vi "Pick_Vitreous.vi"() -> ()   [LabVIEW 2022 SP3]
uses:
  ViewData/-ReadEye/Header.ctl
  ViewData/-ReadEye/TypeDefs/TypeofMean.ctl
  <vilib>/Utility/file.llb/Write Delimited Spreadsheet (string).vi
  <vilib>/Utility/file.llb/Write Delimited Spreadsheet (I64).vi
  <vilib>/Analysis/NI_AALPro.lvlib
panel:
  out "RF":dbl[](graph)
  out "x/y":dbl
  in  "dB":dbl(slide)=-50.20408163265306 scale=0.0..255.0
  out "Waveform Graph":dbl[](graph)
  out "Transducer":u16(ring)=1500 items=["Aviso B10/B15"=1024, "B15 Orbit/Long Vitreous (60 mm)"=1500, "B15 Eye/Vitreous (40 mm)"=2133, "Annular Array"=3282, "Annular Array"=3362, "Lin50"=1000]
  in  "File Params?":bool=TRUE
  out "inc x (mm)":dbl format="%.3f"
  out "inc y (mm)":dbl format="%.3f"
  out "Sector view":dbl[][](graph)
  in  "Pixels in x":i16=256
  in  "Pixels in y":i16=489
  in  "Create EYE batch":bool
  in  "Save Comment ?":bool
  in  "Comment Field (Optional)":string
  in  "Good Case":bool
  in  "Current Image #":i32(slide) min=0 max=134 step=1 scale=0.0..7.0
  in  "stop":bool
  in  "File to Process":path=path "Select a file."
  out "Raw Image File":dbl[][](graph)
  in  "RF lines":i32=170
  in  "RF pts":i32=1024
  out "Total Raw File Size":i32
  out "# Images":dbl
  # "For screening *.raw and *.rf  stacks from Quantel Machines. Attempts to extract info from file name but may need to modify parameters"
  # "Image Parameters"
  # "These remain static!!!"
  # "Push folder symbol (above) to select raw data file to process\nPress \"Page Up\" on keybard to increment up one image\nPress \"Page Down\" on keyboard to decrement down one image\nPress \"ESC\" on keyboard to log number of good image\nSelect \"Save Comment\" to save any text that is entered into \"Comment Field\"\nExit program by pressing \"Stop\""
  # "-\tFor 20MHz, the sampling rate is 60MHz,\n-\tFor 15MHz, depending of the mode:\no\tFor Orbit and Long Vitreous (image displayed with 60mm), the sampling frequency is 20MHz,\no\tFor Eye and Vitreous, (image displayed with 40mm), the sampling frequency is 40MHz\n-\tFor 50MHz, the sampling rate is 80MHz,"
  # "Select  \"Show Context Help\" under \"Help\" menu and scroll over control to see a brief description in pop-up window."
  # "© 2022 Weill Cornell Medicine"
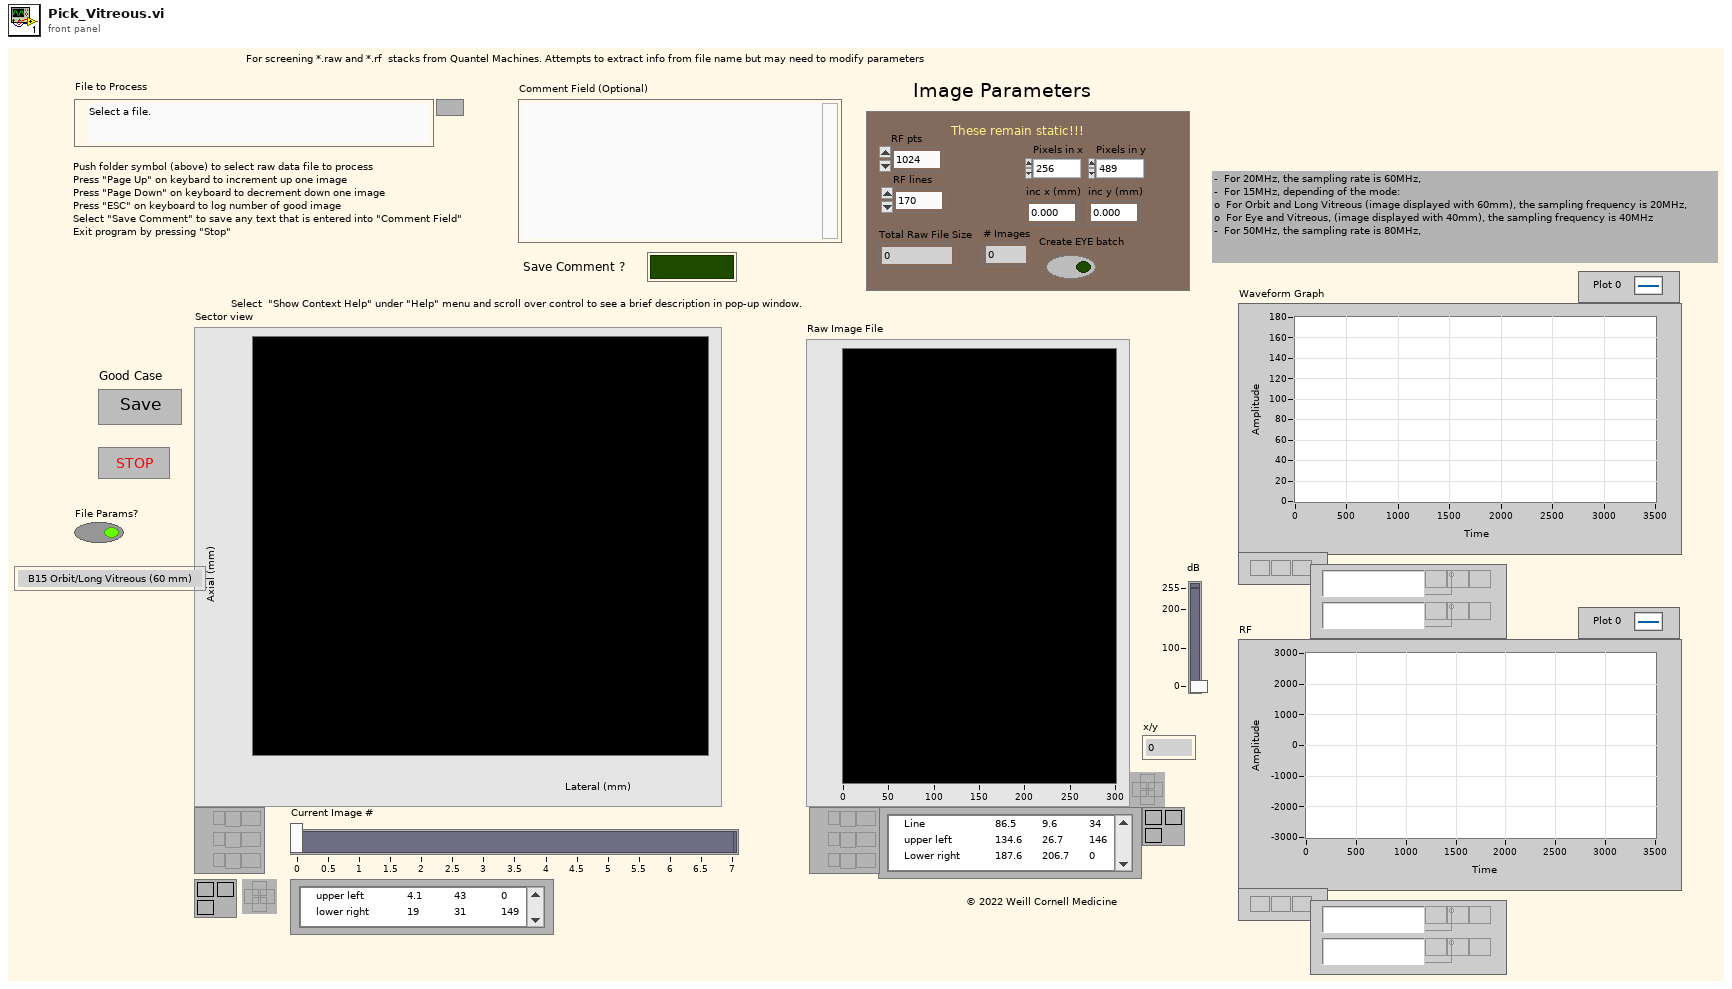
[diagram p1: front panel]
types:
  T1 = typedef "Header.ctl" = cluster{"header info":cluster{"Header":string, "Head length":i16}, "A/D info":cluster{"# rf points per line":u16, "# lines per scan":u16, "sample rate MHz":u16, "# A/D bits":i16, "# bytes per A/D":u16, "TGC Flag":u16, "A/D Type":string}, "Tranducer Info":cluster{"bandwidth":sgl, "center freq":sgl, "start freq":sgl, "ID":i32}, "Scan Info":cluster{"delay":sgl, "pivot distance":sgl, "sector scan angle":sgl, "operator":string, "Scan Mode":string, "location":string}, "Time/Date Info":cluster{"date":string, "time":string}, "RF Info":cluster{"RF file name":string, "RF file att":string, "RF cal file name":string, "RF cal file att":string}, "Patient Info":cluster{"ID":string, "extended ID":string, "age":u16, "sex":string, "previously\nscanned":string, "PSA":sgl, "LOS":u8, "Ethnicty 2":u8, "Race":u8}, "Tissue Type":cluster{"organ":i16, "disease type":i16, "disease location":i16, "IQ_pts":u16, "RcvBuffer":u8, "RcvFrame":u16, "IQBuff":u8, "IQFrame":u16, "IQPage":u8}, "Votage scaling":cluster{"Digitizer (dB)":sgl, "Gain (dB)":sgl, "Atten (dB)":sgl}, "Comment":string, "Misc Info":cluster{"avg num":u16, "c speed":i16, "Div By or SF zones":i16, "XMIT CHS":u8, "RCV CHS":u8, "Xmit angle":sgl}, "Therapy Parameters":cluster{"Theraputic Freq (MHz)":sgl, "Time on (s)":sgl, "Therapy amplitude (mV)":sgl, "Lines Before":u16, "Lines After":u16}, "Scan Settings":cluster{"Energy (uJ or V)":u8, "Damp (Ohm) or Fc":u8, "HP Filt (KHz)":u8, "LP Filt (MHz)":u8, "Gain (db)":u8, "prf (kHz)":sgl, "Distance between\nscan lines (um)":u16, "Distance between\nscan planes (um)":u16, "Scan line gap (um)":sgl, "Scan plane gap (um)":sgl}, "Compression Parameters":cluster{"F1 (MHz)":sgl, "F2 (MHz)":sgl, "% taper":sgl, "duration":sgl}, "Patient Info Xtra":cluster{"First Name":string, "Last Name":string, "Notes":string}, "ROI Box":u16[]}
  T2 = cluster{"low cutoff":i32, "order":i32, "high cutoff":i32}
  T3 = typedef "TypeofMean.ctl" = enum16{"Mean from lines", "Mean just lines", "Poly Mean", "No mean", "Filter"}
  T4 = enum16{"open", "replace", "create", "open or create", "replace or create", "replace or create with confirmation"}
  T5 = cluster{"Frames":i32, "RF Points":i32, "RF lines":i32, "Month":string, "Day":i32, "Year":i32, "Case":string, "data format":string}
  T6 = cluster{"delay":sgl, "pivot distance":sgl, "sector scan angle":sgl, "operator":string, "Scan Mode":string, "location":string}
  T7 = cluster{"X right":dbl, "X left":dbl, "Y low":dbl, "Y high":dbl}
  T8 = typedef "LVPointDoubleTypeDef.ctl" = cluster{"Cursor X":dbl, "Cursor Y":dbl}
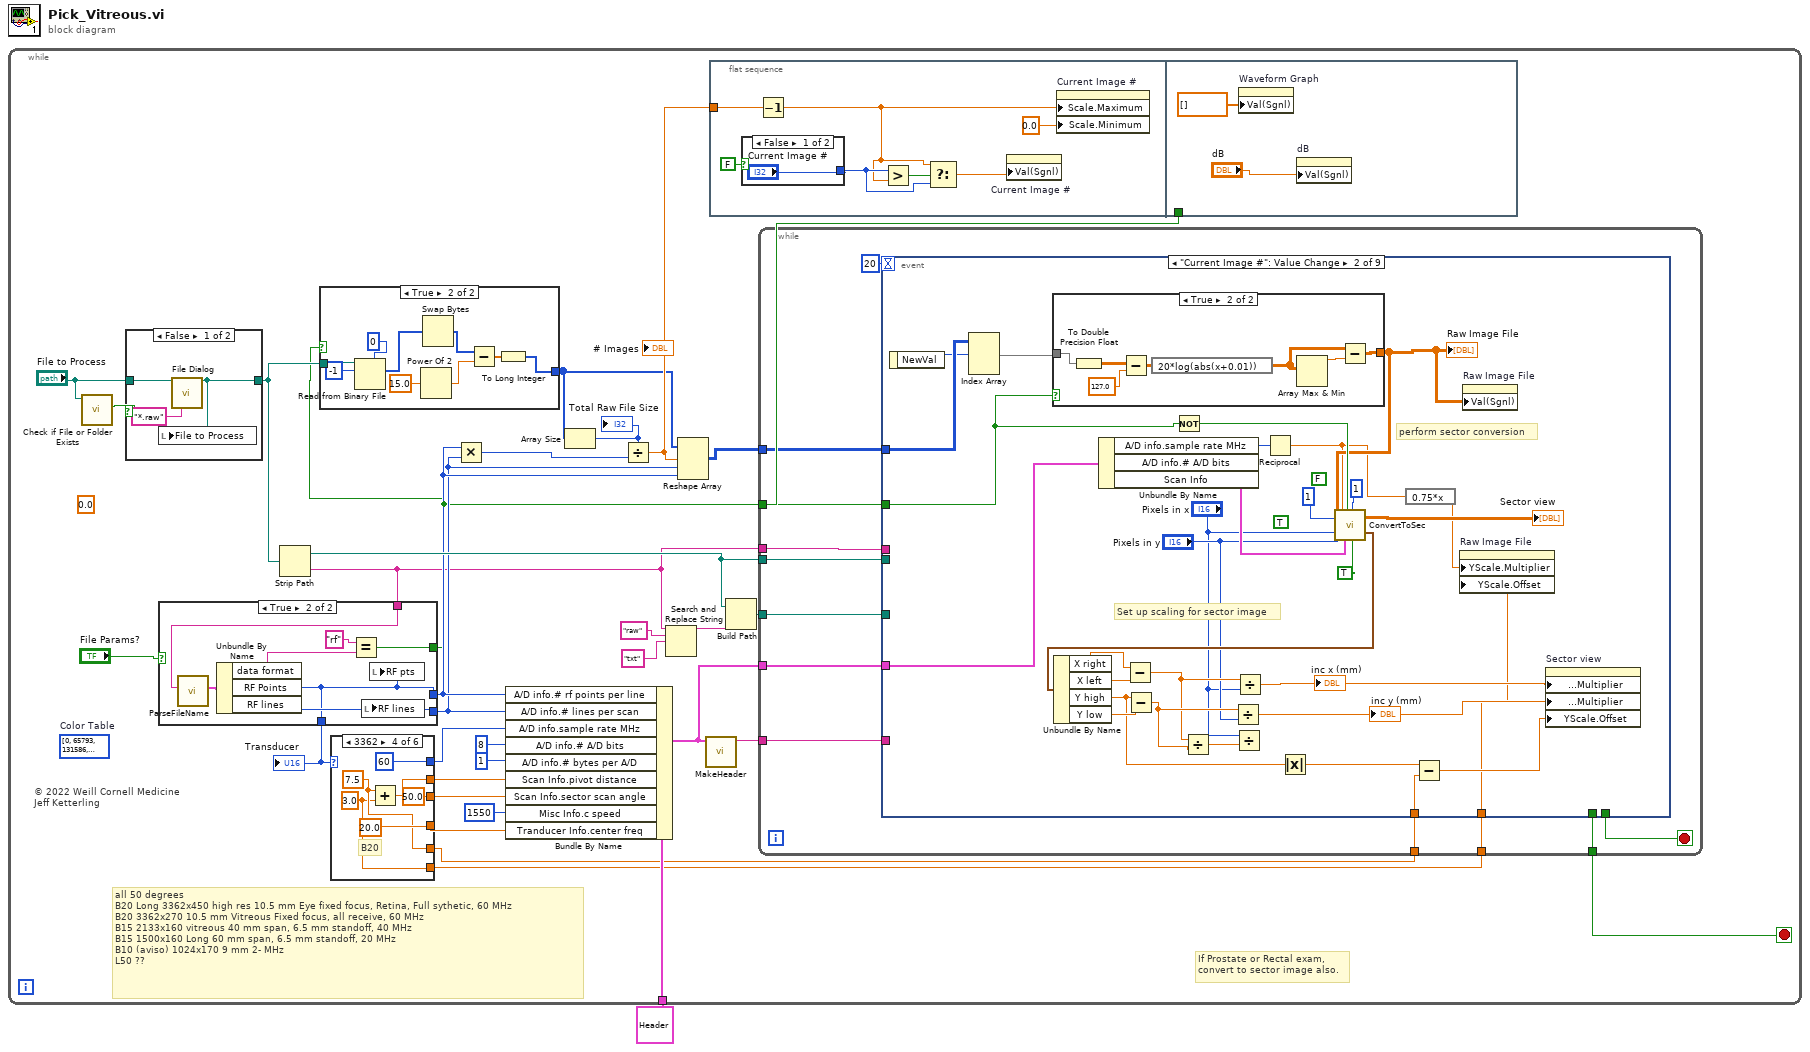
[diagram p0: block diagram]
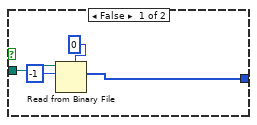
[diagram p2: hidden frame]
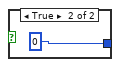
[diagram p3: hidden frame]
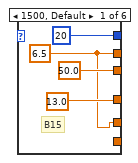
[diagram p4: hidden frame]
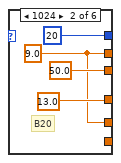
[diagram p5: hidden frame]
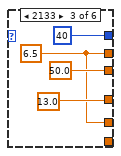
[diagram p6: hidden frame]
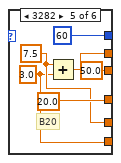
[diagram p7: hidden frame]
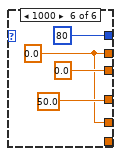
[diagram p8: hidden frame]
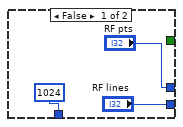
[diagram p9: hidden frame]
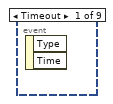
[diagram p11: hidden frame]
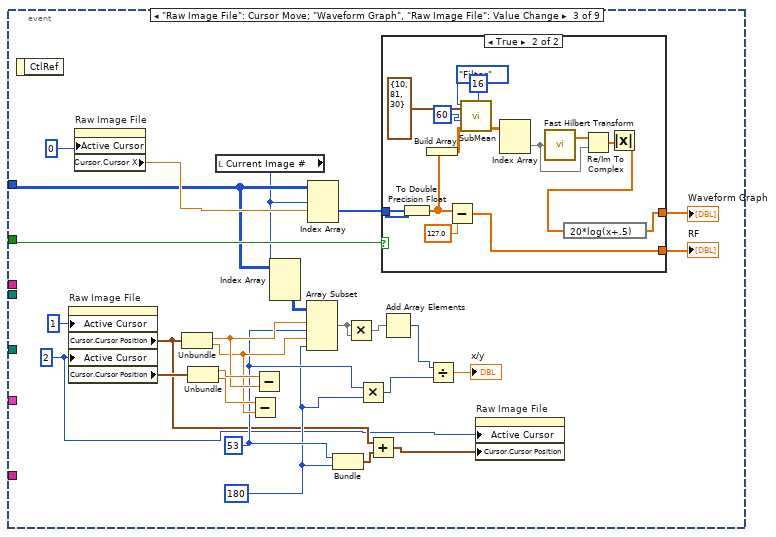
[diagram p13: hidden frame]
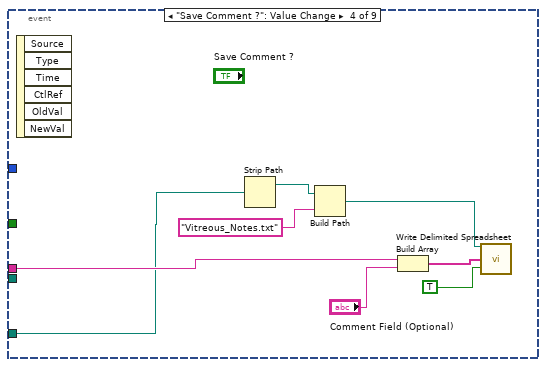
[diagram p15: hidden frame]
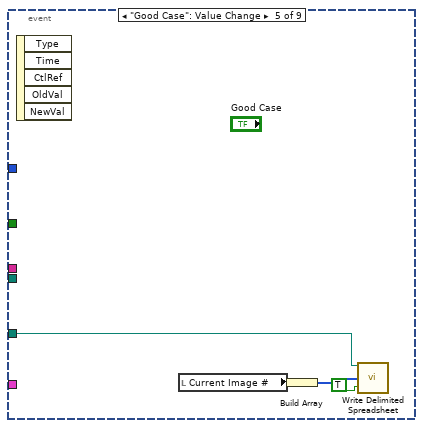
[diagram p16: hidden frame]
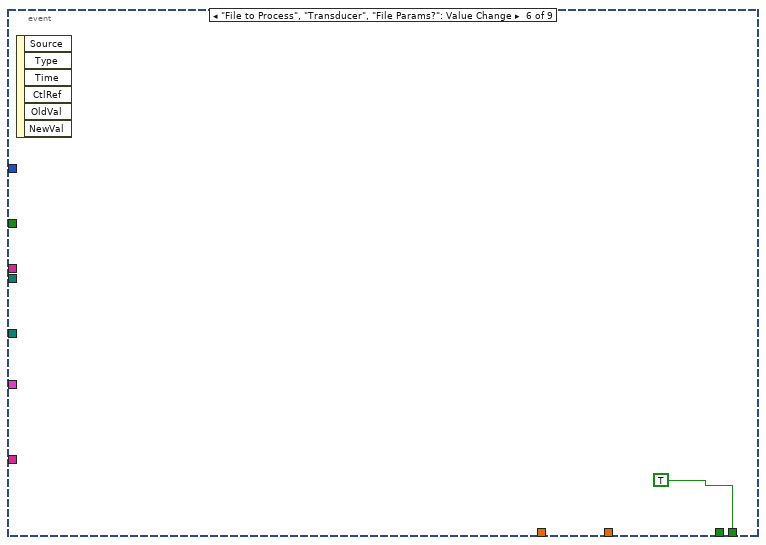
[diagram p17: hidden frame]
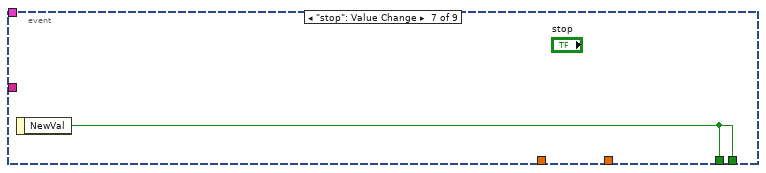
[diagram p18: hidden frame]
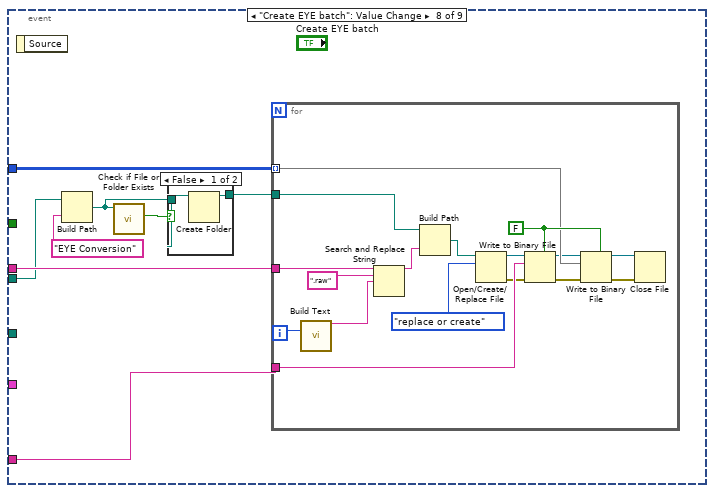
[diagram p19: hidden frame]
diagram:
  n1 = while {
    tunnel: T1 {"header info"={"Header"="", "Head length"=1024}, "A/D info"={"# rf points per line"=0, "# lines per scan"=0, "sample rate MHz"=0, "# A/D bits"=0, "# bytes per A/D"=0, "TGC Flag"=0, "A/D Type"=""}, "Tranducer Info"={"bandwidth"=0.0, "center freq"=0.0, "start freq"=0.0, "ID"=0}, "Scan Info"={"delay"=0.0, "pivot distance"=0.0, "sector scan angle"=0.0, "operator"="", "Scan Mode"="", "location"=""}, "Time/Date Info"={"date"="", "time"=""}, "RF Info"={"RF file name"="", "RF file att"="", "RF cal file name"="", "RF cal file att"=""}, "Patient Info"={"ID"="", "extended ID"="", "age"=0, "sex"="", "previously\nscanned"="", "PSA"=0.0, "LOS"=1, "Ethnicty 2"=3, "Race"=3}, "Tissue Type"={"organ"=0, "disease type"=0, "disease location"=0, "IQ_pts"=0, "RcvBuffer"=0, "RcvFrame"=0, "IQBuff"=0, "IQFrame"=0, "IQPage"=0}, "Votage scaling"={"Digitizer (dB)"=0.0, "Gain (dB)"=0.0, "Atten (dB)"=0.0}, "Comment"="", "Misc Info"={"avg num"=0, "c speed"=0, "Div By or SF zones"=0, "XMIT CHS"=0, "RCV CHS"=0, "Xmit angle"=0.0}, "Therapy Parameters"={"Theraputic Freq (MHz)"=0.1, "Time on (s)"=1.0, "Therapy amplitude (mV)"=50.0, "Lines Before"=20, "Lines After"=80}, "Scan Settings"={"Energy (uJ or V)"=0, "Damp (Ohm) or Fc"=0, "HP Filt (KHz)"=0, "LP Filt (MHz)"=0, "Gain (db)"=0, "prf (kHz)"=0.0, "Distance between\nscan lines (um)"=0, "Distance between\nscan planes (um)"=0, "Scan line gap (um)"=0.0, "Scan plane gap (um)"=0.0}, "Compression Parameters"={"F1 (MHz)"=0.0, "F2 (MHz)"=0.0, "% taper"=0.0, "duration"=0.0}, "Patient Info Xtra"={"First Name"="", "Last Name"="", "Notes"=""}, "ROI Box"=[0, 0, 0, 0]} ("Header In") -> [w25]
    stop <- w30 stop-if-true
    (unwired) u32[] [0, 65793, 131586, 197379, 263172, 328965, 394758, 460551, 526344, 592137, 592137, 657930, 723723, 789516, 855309, 921102, 986895, 1052688, 1118481, 1184274, 1250067, 1315860, 1381653, 1447446, 1513239, 1579032, 1644825, 1710618, 1776411, 1842204, 1907997, 1973790, 2039583, 2105376, 2171169, 2236962, 2302755, 2368548, 2434341, 2500134, 2565927, 2631720, 2697513, 2763306, 2829099, 2894892, 2960685, 3026478, 3092271, 3158064, 3223857, 3289650, 3355443, 3421236, 3487029, 3552822, 3618615, 3684408, 3750201, 3815994, 3881787, 3947580, 4013373, 4079166, 4144959, 4210752, 4276545, 4342338, 4408131, 4473924, 4539717, 4605510, 4671303, 4737096, 4802889, 4868682, 4934475, 5000268, 5066061, 5131854, 5197647, 5263440, 5329233, 5395026, 5460819, 5526612, 5592405, 5658198, 5723991, 5789784, 5855577, 5921370, 5987163, 6052956, 6118749, 6184542, 6250335, 6316128, 6381921, 6447714, 6513507, 6579300, 6645093, 6710886, 6776679, 6842472, 6908265, 6974058, 7039851, 7105644, 7171437, 7237230, 7303023, 7368816, 7434609, 7500402, 7566195, 7631988, 7697781, 7763574, 7829367, 7895160, 7960953, 8026746, 8092539, 8158332, 8224125, 8289918, 8355711, 8421504, 8487297, 8553090, 8618883, 8684676, 8750469, 8816262, 8882055, 8947848, 9013641, 9079434, 9145227, 9211020, 9276813, 9342606, 9408399, 9474192, 9539985, 9605778, 9671571, 9737364, 9803157, 9868950, 9934743, 10000536, 10066329, 10132122, 10197915, 10263708, 10329501, 10395294, 10461087, 10526880, 10592673, 10658466, 10724259, 10790052, 10855845, 10921638, 10987431, 11053224, 11119017, 11184810, 11250603, 11316396, 11382189, 11447982, 11513775, 11579568, 11645361, 11711154, 11776947, 11842740, 11908533, 11974326, 12040119, 12105912, 12171705, 12237498, 12303291, 12369084, 12434877, 12500670, 12566463, 12632256, 12698049, 12763842, 12829635, 12895428, 12961221, 13027014, 13092807, 13158600, 13224393, 13290186, 13355979, 13421772, 13487565, 13553358, 13619151, 13684944, 13750737, 13816530, 13882323, 13948116, 14013909, 14079702, 14145495, 14211288, 14277081, 14342874, 14408667, 14474460, 14540253, 14606046, 14671839, 14737632, 14803425, 14869218, 14935011, 15000804, 15066597, 15132390, 15198183, 15263976, 15329769, 15395562, 15461355, 15527148, 15592941, 15658734, 15724527, 15790320, 15856113, 15921906, 15987699, 16053492, 16119285, 16185078, 16250871, 16316664, 16382457, 16448250, 16514043, 16579836, 16645629, 0]  # Color Table
    (unwired) sgl 0.0 ("Scan Info.pivot distance")
    # "If Prostate or Rectal exam,\nconvert to sector image also."
    # "all 50 degrees\nB20 Long 3362x450 high res 10.5 mm Eye fixed focus, Retina, Full sythetic, 60 MHz\nB20 3362x270 10.5 mm Vitreous Fixed focus, all receive, 60 MHz\nB15 2133x160 vitreous 40 mm span, 6.5 mm standoff, 40 MHz\nB15 1500x160 Long 60 mm span, 6.5 mm standoff, 20 MHz \nB10 (aviso) 1024x170 9 mm 2- MHz\nL50 ??"
    # "© 2022 Weill Cornell Medicine\nJeff Ketterling"
    n2 = call <vilib>:"Check if File or Folder Exists.vi"("path"="File to Process") -> ("file or folder exists?"=w21:bool)  [unwired: 8 in, 2 out]
    n3 = case shown="False" w21 {
      tunnel: [w97 w99] -> w19
      tunnel: "File to Process" -> [w98 w99]
      frame False {
        n4 = call "File Dialog"("start path"=w98, "pattern (all files)"="*.raw") -> ("selected path"=w97:path)  [unwired: 10 in, 3 out]
        n5 = local write "File to Process"(w97) -> ()
      }
      frame True {
      }
    }
    n6 = Strip Path(path=w19) -> (stripped path=w23:path, name=w14:string)
    n7 = case shown="True" "File Params?" {
      tunnel: ["RF pts" w89] -> w18
      tunnel: ["RF lines" w93] -> w17
      tunnel: w14 -> [_ w94]
      tunnel: [_ w90] -> w5
      tunnel: [1024 ("RF Points") w89] -> w7
      frame False {
      }
      frame True {
        n8 = call "ParseFileName.vi"("Quantel File Name"=w94) -> ("File Parameters"=w95:T5)  [unwired: 10 in]
        n9 = Unbundle By Name(w95) -> ("data format"=w92:string, "RF Points"=w89:i32, "RF lines"=w93:i32)
        n10 = Equal?(x="rf", y=w92) -> (x = y?=w90:bool)
        n11 = local write "RF lines"(w93) -> ()
        n12 = local write "RF pts"(w89) -> ()
      }
    }
    "Transducer" <- w7
    n13 = case shown="True" w5 {
      tunnel: [w34 w38] -> w4
      tunnel: w19 -> [w36 w44]
      frame False {
        n14 = Read from Binary File(5:u8 0, 10:-1 ("count (1)"), 11:w36) -> (2:w34:u8[])  [unwired: 3 in, 3 out]
      }
      frame True {
        n15 = Read from Binary File(5:u16 0, 10:-1 ("count (1)"), 11:w44) -> (2:w40:u16[])  [unwired: 3 in, 3 out]
        n16 = Power Of 2(x=15.0) -> (2^x=w42:dbl)
        n17 = Swap Bytes(anything=w40) -> (byte swapped=w43:u16[])
        n18 = Subtract(x=w43, y=w42) -> (x-y=w39:dbl[])
        n19 = To Long Integer(number=w39) -> (32bit integer=w38:i32[])
      }
    }
    n20 = case shown="3362" w7 {
      tunnel: [sgl 13.0 ("Tranducer Info.center freq") sgl 13.0 ("Tranducer Info.center freq") sgl 13.0 ("Tranducer Info.center freq") sgl 20.0 ("Tranducer Info.center freq") sgl 20.0 ("Tranducer Info.center freq") sgl 50.0 ("Tranducer Info.center freq")] -> w11
      tunnel: [sgl 50.0 ("Scan Info.sector scan angle") sgl 50.0 ("Scan Info.sector scan angle") sgl 50.0 ("Scan Info.sector scan angle") sgl 50.0 ("Scan Info.sector scan angle") sgl 50.0 ("Scan Info.sector scan angle") sgl 0.0 ("Scan Info.sector scan angle")] -> w9
      tunnel: [w58 w62 w66 w72 w78 w82] -> w8
      tunnel: [u16 20 ("A/D info.sample rate MHz") u16 20 ("A/D info.sample rate MHz") u16 40 ("A/D info.sample rate MHz") u16 60 ("A/D info.sample rate MHz") u16 60 ("A/D info.sample rate MHz") u16 80 ("A/D info.sample rate MHz")] -> w10
      tunnel: [w58 w62 w66 w71 w77 w82] -> w3
      tunnel: [_ _ _ w70 w76 _] -> w2
      frame 1500, Default {
        w58 = sgl 6.5 ("Scan Info.pivot distance")
        # "B15"
      }
      frame 1024 {
        w62 = sgl 9.0 ("Scan Info.pivot distance")
        # "B20"
      }
      frame 2133 {
        w66 = sgl 6.5 ("Scan Info.pivot distance")
      }
      frame 3362 {
        w70 = sgl 3.0 ("y")
        w71 = sgl 7.5 ("Scan Info.pivot distance")
        # "B20"
        n21 = Add(x=w71, y=w70) -> (x+y=w72:sgl)
      }
      frame 3282 {
        w76 = sgl 3.0 ("y")
        w77 = sgl 7.5 ("Scan Info.pivot distance")
        # "B20"
        n22 = Add(x=w77, y=w76) -> (x+y=w78:sgl)
      }
      frame 1000 {
        w82 = sgl 0.0 ("Scan Info.pivot distance")
      }
    }
    n23 = Multiply(x=w18, y=w17) -> (x*y=w32:i32)
    n24 = Bundle By Name(cluster=w25, "A/D info.# rf points per line"=w18, "A/D info.# lines per scan"=w17, "A/D info.sample rate MHz"=w10, "A/D info.# A/D bits"=i16 8, "A/D info.# bytes per A/D"=u16 1, "Scan Info.pivot distance"=w8, "Scan Info.sector scan angle"=w9, "Misc Info.c speed"=i16 1550, "Tranducer Info.center freq"=w11) -> (w22:T1)
    n25 = Array Size(array=w4) -> (size(s)=w33:i32)
    "Total Raw File Size" <- w33
    n26 = Divide(x=w33, y=w32) -> (x/y=w6:dbl)
    "# Images" <- w6
    n27 = Search and Replace String(input string=w14, search string="raw", replace string="txt" ("replace string (\"\")")) -> (result string=w27:string)  [unwired: 5 in, 3 out]
    n28 = Reshape Array(w4, w6, w17, w18) -> (w31:i32[][][])
    n29 = call "MakeHeader.vi"("Header In"=w22) -> ("Header String"=w24:string)  [unwired: 6 out]
    n30 = flat-sequence {
      tunnel: w6 -> [w48]
      tunnel: w5 -> [_]
      frame #0 {
        n31 = case shown="False" FALSE {
          tunnel: ["Current Image #" 0 ("Value (Signaling)")] -> w50
          frame False {
          }
          frame True {
          }
        }
        n32 = Decrement(x=w48) -> (x-1=w47:dbl)
        n33 = Greater?(x=w50, y=w47) -> (0:w51:bool)
        n34 = Select(t=w47, s=w51, f=w50) -> (s? t:f=w49:dbl)
        n35 = property on="Current Image #" class="Slide (strict)"("Val(Sgnl)"=w49) -> ()  [unwired: 2 in, 2 out]
        n36 = property on="Current Image #" class="Slide (strict)"("Scale.Maximum"=w47, "Scale.Minimum"=0.0 ("Scale.Range:Minimum")) -> ()  [unwired: 2 in, 2 out]
      }
      frame #1 {
        n37 = property on="Waveform Graph" class="WFGraph (strict)"("Val(Sgnl)"=dbl[] [] ("Value (Signaling)")) -> ()  [unwired: 2 in, 2 out]
        n38 = property on="dB" class="Slide (strict)"("Val(Sgnl)"="dB") -> ()  [unwired: 2 in, 2 out]
      }
    }
    n39 = Build Path(base path=w23, name or relative path=w27) -> (appended path=w26:path)
    n40 = while {
      tunnel: w31 -> [w111]
      tunnel: [w108] -> w30
      tunnel: w26 -> [w107]
      tunnel: w14 -> [w106]
      tunnel: w24 -> [w105]
      tunnel: w23 -> [w104]
      tunnel: w22 -> [w103]
      tunnel: w5 -> [w102]
      tunnel: w3 -> [w101]
      tunnel: w2 -> [w100]
      stop <- w109 stop-if-true
      n41 = event shown="[1] \"Current Image #\": Value Change" {
        selector: _ -> [_ _ _ _ _ _ _ _ _]
        dyn-events: _ -> [_ _ _ _ _ _ _ _ _]
        timeout: 20 -> [_ _ _ _ _ _ _ _ _]
        tunnel: w111 -> [_ w142 w167 _ _ _ _ w214 _]
        tunnel: [_ _ _ _ _ TRUE ("NewVal") w206 _ _] -> w109
        tunnel: [_ _ _ _ _ _ w206 _ _] -> w108
        tunnel: w107 -> [_ _ _ w197 w201 _ _ _ _]
        tunnel: w106 -> [_ _ _ w200 _ _ _ w212 _]
        tunnel: w105 -> [_ _ _ _ _ _ _ w213 _]
        tunnel: w104 -> [_ _ _ _ _ _ _ w211 _]
        tunnel: w103 -> [_ w124 _ _ _ _ _ _ _]
        tunnel: w102 -> [_ w121 w175 _ _ _ _ _ w238]
        tunnel: w101 -> [_ w116 _ _ _ _ _ _ _]
        tunnel: w100 -> [_ w114 _ _ _ _ _ _ _]
        event Timeout {
          n42 = event-data() -> ()  [unwired: 1 in, 2 out]
        }
        event "Current Image #": Value Change {
          (unwired) FALSE ("Abs?")
          (unwired) TRUE ("no oversample?")
          # "Set up scaling for sector image"
          # "perform sector conversion"
          n43 = event-data() -> ("NewVal"=w141:i32)  [unwired: 1 in]
          n44 = Index Array(array=w142, index (dim 0)=w141) -> (element=w123:i32[][])  [unwired: 2 in]
          n45 = case shown="True" w121 {
            tunnel: w123 -> [w143 w146]
            tunnel: [w143 w148] -> w119
            frame False {
            }
            frame True {
              n46 = To Double Precision Float(number=w146) -> (double precision float=w145:dbl[][])
              n47 = Subtract(x=w145, y=127.0) -> (x-y=w144:dbl[][])
              n48 = expression code="20*log(abs(x+0.01))"(w144) -> (w150:dbl[][])
              n49 = Array Max & Min(array=w150) -> (max value=w149:dbl)  [unwired: 3 out]
              n50 = Subtract(x=w150, y=w149) -> (x-y=w148:dbl[][])
            }
          }
          "Raw Image File" <- w119
          n51 = Unbundle By Name(w124) -> ("A/D info.sample rate MHz"=w139:u16, "Scan Info"=w138:T6)  [unwired: 1 out]
          n52 = Not(x=w121) -> (.not. x?=w120:bool)
          n53 = Reciprocal(x=w139) -> (1/x=w112:dbl)
          n54 = call "ConvertToSec.vi"("raw image data in"=w119, "reduce pts by factor of"=1, "pixels in x"="Pixels in x", "pixels in y"="Pixels in y", "Time between rf pts\nmicros"=w112, "Scan Info"=w138, "Abs?"=w120, "Smooth factor"=1, "use min z value?"=TRUE) -> ("raw sector out"=→"Sector view":dbl[][], "Axis scaling Params"=w128:T7)  [unwired: 3 in, 6 out]
          n55 = Unbundle By Name(w128) -> ("X right"=w136:dbl, "X left"=w134:dbl, "Y high"=w118:dbl, "Y low"=w135:dbl)
          n56 = Subtract(x=w136, y=w134) -> (x-y=w131:dbl)
          n57 = Subtract(x=w118, y=w135) -> (x-y=w133:dbl)
          n58 = Divide(x=w131, y=w133) -> (x/y=w132:dbl)
          n59 = Divide(x=w133, y="Pixels in y") -> (x/y=w129:dbl)
          "inc y (mm)" <- w129
          n60 = Divide(x="Pixels in x", y=w132) -> ()  [unwired: 1 out]
          n61 = Divide(x=w131, y="Pixels in x") -> (x/y=w130:dbl)
          "inc x (mm)" <- w130
          n62 = Absolute Value(x=w118) -> (abs(x)=w117:dbl)
          n63 = expression code="0.75*x"(w112) -> (w113:dbl)
          n64 = Subtract(x=w117, y=w116) -> (x-y=w115:dbl)
          n65 = property on="Raw Image File" class="IntGraph (strict)"("YScale.Multiplier"=w113, "YScale.Offset"=w114) -> ()  [unwired: 2 in, 2 out]
          n66 = property on="Raw Image File" class="IntGraph (strict)"("Val(Sgnl)"=w119) -> ()  [unwired: 2 in, 2 out]
          n67 = property on="Sector view" class="IntGraph (strict)"("X Scale.Offset and Multiplier:Multiplier"=w130, "Y Scale.Offset and Multiplier:Multiplier"=w129, "YScale.Offset"=w115) -> ()  [unwired: 2 in, 2 out]
        }
        event "Raw Image File": Cursor Move; "Waveform Graph", "Raw Image File": Value Change {
          w156 = 180
          w157 = 53
          w152 = u32 2 ("Active Cursor")
          n68 = event-data() -> ()  [unwired: 1 in, 1 out]
          n69 = property on="Raw Image File" class="IntGraph (strict)"("Active Cursor"=u32 1, "Active Cursor"=w152) -> ("Cursor.Cursor Position"=w154:T8, "Cursor.Cursor Position"=w170:T8)  [unwired: 2 in, 2 out]
          n70 = property on="Raw Image File" class="IntGraph (strict)"("Active Cursor"=u32 0) -> ("Cursor.Cursor X"=w173:dbl)  [unwired: 2 in, 2 out]
          n71 = Unbundle(w154) -> ("Cursor X"=w164:dbl, "Cursor Y"=w163:dbl)
          n72 = Unbundle(w170) -> ("Cursor X"=w169:dbl, "Cursor Y"=w168:dbl)
          n73 = local read "Current Image #"() -> (w166:i32)
          n74 = Subtract(x=w168, y=w163) -> ()  [unwired: 1 out]
          n75 = Subtract(x=w169, y=w164) -> ()  [unwired: 1 out]
          n76 = Index Array(array=w167, index (dim 0)=w166) -> (element=w165:i32[][])  [unwired: 2 in]
          n77 = Array Subset(array=w165, index (row)=w164, length (row)=w157, index (col)=w163, length (col)=w156) -> (w159:i32[][])
          n78 = Index Array(array=w167, index (dim 0)=w166, index (dim 1)=w173) -> (element=w176:i32[])  [unwired: 1 in]
          n79 = Bundle(w157, w156) -> (w155:cluster{i32, i32})  [unwired: 1 in]
          n80 = Multiply(x=w159, y=w159) -> (x*y=w158:i32[][])
          n81 = Multiply(x=w157, y=w156) -> (x*y=w162:i32)
          n82 = Add(x=w154, y=w155) -> (x+y=w153:T8)
          n83 = case shown="True" w175 {
            tunnel: w176 -> [w177 w191]
            tunnel: [w177 w188] -> w174
            tunnel: [_ w187] -> w151
            frame False {
            }
            frame True {
              n84 = To Double Precision Float(number=w191) -> (double precision float=w182:dbl[])
              n85 = Build Array(w182) -> (w186:dbl[][])
              n86 = Subtract(x=w182, y=127.0) -> (x-y=w187:dbl[])
              n87 = call "SubMean.vi"("Bit Depth"=16, "Scan Data In"=w186, "Samp Rate (MHz)"=i16 60, "Filter Prams"=T2 {"low cutoff"=10, "order"=81, "high cutoff"=30}, "Type of Mean"=TypeofMean."Filter") -> ("Array"=w183:dbl[][])  [unwired: 1 in, 2 out]
              n88 = Index Array(array=w183) -> (element=w181:dbl[])  [unwired: 2 in]
              n89 = call <vilib>:"Fast Hilbert Transform.vi"("X"=w181) -> ("Hilbert{X}"=w190:dbl[])  [unwired: 1 out]
              n90 = Re/Im To Complex(1:w181, 2:w190) -> (0:w189:cdb[])
              n91 = Absolute Value(x=w189) -> (abs(x)=w178:dbl[])
              n92 = expression code="20*log(x+.5)"(w178) -> (w188:dbl[])
            }
          }
          "Waveform Graph" <- w174
          "RF" <- w151
          n93 = Add Array Elements(numeric array=w158) -> (sum=w161:i32)
          n94 = Divide(x=w161, y=w162) -> (x/y=→"x/y":dbl)
          n95 = property on="Raw Image File" class="IntGraph (strict)"("Active Cursor"=w152, "Cursor.Cursor Position"=w153) -> ()  [unwired: 2 in, 2 out]
        }
        event "Save Comment ?": Value Change {
          n96 = event-data() -> ()  [unwired: 1 in, 6 out]
          n97 = Strip Path(path=w197) -> (stripped path=w196:path)  [unwired: 1 out]
          n98 = Build Path(base path=w196, name or relative path="Vitreous_Notes.txt" ("search string")) -> (appended path=w194:path)
          n99 = Build Array(w200, "Comment Field (Optional)") -> (w193:string[])
          n100 = call-poly <vilib>:"Write Delimited Spreadsheet.vi"("file path (dialog if empty)"=w194, "1D data"=w193, "transpose? (no:F)"=TRUE ("append to file? (new file:F)")) -> ()  [unwired: 11 in, 2 out]
        }
        event "Good Case": Value Change {
          n101 = event-data() -> ()  [unwired: 1 in, 5 out]
          n102 = local read "Current Image #"() -> (w203:i32)
          n103 = Build Array(w203) -> (w202:i32[])
          n104 = call-poly <vilib>:"Write Delimited Spreadsheet.vi"("file path (dialog if empty)"=w201, "1D data"=w202, "transpose? (no:F)"=TRUE ("append to file? (new file:F)")) -> ()  [unwired: 11 in, 2 out]
        }
        event "File to Process", "Transducer", "File Params?": Value Change {
          n105 = event-data() -> ()  [unwired: 1 in, 6 out]
        }
        event "stop": Value Change {
          n106 = event-data() -> ("NewVal"=w206:bool)  [unwired: 1 in]
        }
        event "Create EYE batch": Value Change {
          n107 = event-data() -> ()  [unwired: 1 in, 1 out]
          n108 = Build Path(base path=w211, name or relative path="EYE Conversion" ("search string")) -> (appended path=w208:path)
          n109 = call <vilib>:"Check if File or Folder Exists.vi"("path"=w208) -> ("file or folder exists?"=w207:bool)  [unwired: 8 in, 2 out]
          n110 = case shown="False" w207 {
            tunnel: [w216 w217] -> w209
            tunnel: w208 -> [w215 w217]
            frame False {
              n111 = Create Folder(path (use dialog)=w215) -> (created path=w216:path)  [unwired: 2 in, 2 out]
            }
            frame True {
            }
          }
          n112 = for {
            tunnel: w214 -> [w232] mode=indexing
            tunnel: w213 -> [w233]
            tunnel: w212 -> [w229]
            tunnel: w209 -> [w218]
            i -> [w227]
            w234 = FALSE ("prepend array or string size? (T)")
            n113 = call "Build Text"("num"=w227) -> ("Result"=w226:string)  [unwired: 13 in, 1 out]
            n114 = Search and Replace String(input string=w229, search string=".raw", replace string=w226) -> (result string=w222:string)  [unwired: 5 in, 3 out]
            n115 = Build Path(base path=w218, name or relative path=w222) -> (appended path=w223:path)
            n116 = Open/Create/Replace File(file path (use dialog)=w223, operation (0:open)=T4."replace or create") -> (refnum out=w224:refnum<file>, error out=w225:errorcluster)  [unwired: 4 in, 1 out]
            n117 = Write to Binary File(file (use dialog)=w224, data=w233, error in=w225, 5:w234) -> (refnum out=w231:refnum<file>, error out=w230:errorcluster)  [unwired: 2 in, 1 out]
            n118 = Write to Binary File(file (use dialog)=w231, data=w232, error in=w230, 5:w234) -> (refnum out=w219:refnum<file>, error out=w220:errorcluster)  [unwired: 2 in, 1 out]
            n119 = Close File(refnum=w219, error in=w220) -> ()  [unwired: 2 out]
          }
        }
        event "dB": Value Change {
          n120 = event-data() -> ("NewVal"=w237:dbl)  [unwired: 1 in, 5 out]
          n121 = case shown="False" w238 {
            tunnel: [0 -60] -> w239
            tunnel: [w242 0] -> w240
            tunnel: w237 -> [w243 w249]
            tunnel: [0.0 ("NewVal") w250] -> w236
            tunnel: [w241 0.0 ("NewVal")] -> w235
            frame False {
              w242 = 255
              n122 = Less Than 0?(x=w243) -> (x < 0?=w244:bool)
              n123 = case shown="True" w244 {
                tunnel: w243 -> [w247 _]
                tunnel: w242 -> [_ w248]
                tunnel: [w247 w248] -> w241
                frame False {
                }
                frame True {
                  n124 = property on="dB" class="Slide (strict)"("Value"=w248) -> ()  [unwired: 2 in, 2 out]
                }
              }
            }
            frame True {
              n125 = Greater Than 0?(x=w249) -> (x > 0?=w251:bool)
              n126 = case shown="False" w251 {
                tunnel: [w255 w256] -> w250
                tunnel: w249 -> [w255 _]
                frame False {
                }
                frame True {
                  w256 = -45
                  n127 = property on="dB" class="Slide (strict)"("Value"=w256) -> ()  [unwired: 2 in, 2 out]
                }
              }
            }
          }
          n128 = property on="Raw Image File" class="IntGraph (strict)"("ZScale.Maximum"=w235, "ZScale.Minimum"=w236) -> ()  [unwired: 2 in, 2 out]
          n129 = property on="dB" class="Slide (strict)"("Scale.Maximum"=w240, "Scale.Minimum"=w239) -> ()  [unwired: 2 in, 2 out]
          n130 = property on="Sector view" class="IntGraph (strict)"("ZScale.Maximum"=w235, "ZScale.Minimum"=w236) -> ()  [unwired: 2 in, 2 out]
        }
      }
    }
  }
